vi "API Parse Response.vi"(7 "PIM.API.Response.Unique":T3) -> (3 "Sample":T1[](array[typedef]), 4 "Action":string, 6 "Double":dbl[](array[numeric]), 8 "Integer":i32[](array[numeric]), 10 "Boolean":bool[](array[boolean]), 14 "error out":errorcluster, 15 "String":string[](array[string]))   [LabVIEW 2011]
uses:
  Controls/PIM.API.Response.Unique.ctl
  Controls/PIM.API.Response.Samples.ctl
  iQA Sweep Behavior.ctl
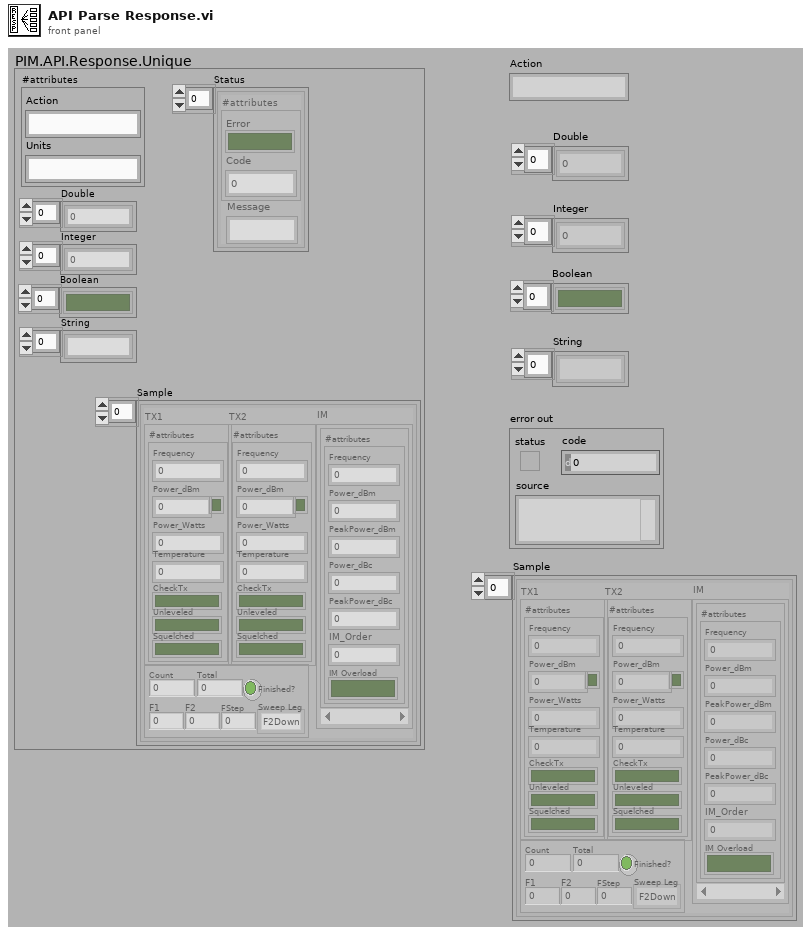
[diagram p1: front panel]
types:
  T1 = typedef "PIM.API.Response.Samples.ctl" = cluster{"TX1":cluster{"#attributes":cluster{"Frequency":dbl, "Power_dBm":dbl, "Power_Watts":dbl, "CheckTx":bool, "Unleveled":bool, "Squelched":bool, "Temperature":dbl, "ToneOn":bool}}, "TX2":cluster{"#attributes":cluster{"Frequency":dbl, "Power_dBm":dbl, "Power_Watts":dbl, "CheckTx":bool, "Unleveled":bool, "Squelched":bool, "Temperature":dbl, "ToneOn":bool}}, "IM":cluster{"#attributes":cluster{"Frequency":dbl, "Power_dBm":dbl, "PeakPower_dBm":dbl, "Power_dBc":dbl, "PeakPower_dBc":dbl, "IM_Order":u8, "IM Overload":bool}}[], "#attributes":cluster{"Count":u32, "Total":u32, "Finished?":bool, "Sweep Leg":T2, "F1":dbl, "F2":dbl, "FStep":dbl}}
  T2 = typedef "iQA Sweep Behavior.ctl" = enum16{"F2Down", "F1Up", "RxMultiIM"}
  T3 = typedef "PIM.API.Response.Unique.ctl" = cluster{"#attributes":cluster{"Action":string, "Units":string}, "Double":dbl[], "Integer":i32[], "Boolean":bool[], "String":string[], "Sample":T1[], "Status":cluster{"#attributes":cluster{"Error":bool, "Code":i32}, "Message":string}[]}
  T4 = cluster{"#attributes":cluster{"Error":bool, "Code":i32}, "Message":string}[]
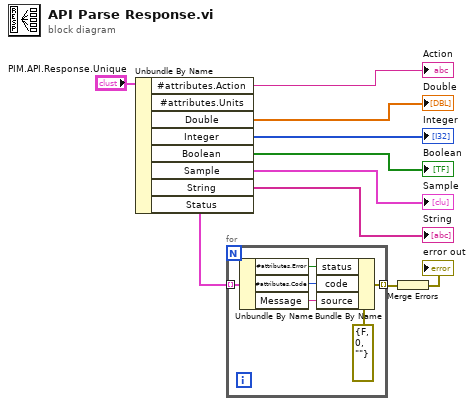
[diagram p0: block diagram]
diagram:
  n1 = Unbundle By Name("PIM.API.Response.Unique") -> ("#attributes.Action"=→"Action":string, "Double"=→"Double":dbl[], "Integer"=→"Integer":i32[], "Boolean"=→"Boolean":bool[], "Sample"=→"Sample":T1[], "String"=→"String":string[], "Status"=w3:T4)  [unwired: 1 out]
  n2 = for {
    tunnel: w3 -> [w12] mode=indexing
    tunnel: [w11] -> w2 mode=indexing
    n3 = Unbundle By Name(w12) -> ("#attributes.Error"=w15:bool, "#attributes.Code"=w14:i32, "Message"=w13:string)
    n4 = Bundle By Name(cluster=errorcluster {"status"=FALSE, "code"=0, "source"=""} ("error out"), "status"=w15, "code"=w14, "source"=w13) -> (w11:errorcluster)
  }
  n5 = Merge Errors(w2) -> (→"error out":errorcluster)
